vi "CoordAxis_S.vi"() -> (3 "out Coordinate Axis":T1)   [LabVIEW 2019, in "Trajectory_Library.lvlib"]
doc: "Returns a coordinate axis corresponding to -X in the NWU coordinate system. (South)\n\nInputs: \n -- none --\n\nOutputs:\n - Coordinate Axis -- A data cluster representing a coordinate system axis with respect to the NWU coordinate system."
uses:
  Trajectory_Library.lvlib
  TypeDef/COORDINATE_AXIS.ctl
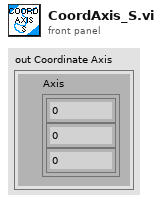
[diagram p1: front panel]
types:
  T1 = typedef "Trajectory_Library.lvlib/COORDINATE_AXIS.ctl" = cluster{"Axis":dbl[]}
  T2 = typedef "WPILib_Math.lvlib/COORDINATE_AXIS.ctl" = cluster{"Axis":dbl[]}
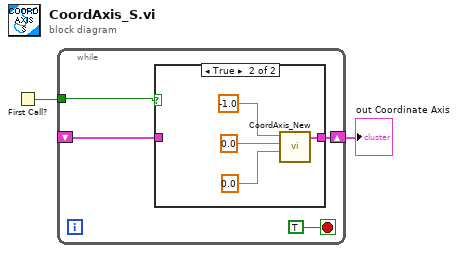
[diagram p0: block diagram]
diagram:
  n1 = First Call?() -> (First Call?: T/F=w1:bool)
  n2 = while {
    shift-right: [w6] -> w2
    shift-left: _ -> [w3]
    tunnel: w1 -> [w4]
    stop <- TRUE stop-if-true
    n3 = case shown="True" w4 {
      tunnel: [w7 w11] -> w6
      tunnel: w3 -> [w7 _]
      frame False {
      }
      frame True {
        n4 = call "CoordAxis_New.vi"("Z"=0.0, "Y"=0.0, "X"=-1.0) -> ("out Coordinate Axis"=w11:T2)  [unwired: 8 in]
      }
    }
  }
  "out Coordinate Axis" <- w2
